vi "HFRR ADV v06 new software.vi"() -> ()   [LabVIEW 2025] (continued)
              n1804 = String Subset(string=w2036, offset (0)=55, length (rest)=9 ("length (rest)")) -> (substring=w2044:string)
              n1805 = String Subset(string=w2036, offset (0)=25) -> (substring=w2040:string)  [unwired: 1 in]
              n1806 = String Subset(string=w2036, offset (0)=15, length (rest)=9 ("length (rest)")) -> (substring=w2065:string)
              n1807 = String Subset(string=w2036, offset (0)=0, length (rest)=14 ("length (rest)")) -> (substring=w2062:string)
              n1808 = String Subset(string=w2036, offset (0)=45, length (rest)=9 ("length (rest)")) -> (substring=w2049:string)
              n1809 = String Subset(string=w2036, offset (0)=65, length (rest)=9 ("length (rest)")) -> (substring=w2055:string)
              n1810 = Fract/Exp String To Number(string=w2038) -> (number=w2035:dbl)  [unwired: 3 in, 1 out]
              n1811 = Fract/Exp String To Number(string=w2059) -> (number=w2057:dbl)  [unwired: 3 in, 1 out]
              n1812 = Fract/Exp String To Number(string=w2044) -> (number=w2042:dbl)  [unwired: 3 in, 1 out]
              n1813 = Fract/Exp String To Number(string=w2040) -> (number=w2039:dbl)  [unwired: 3 in, 1 out]
              n1814 = Fract/Exp String To Number(string=w2065) -> (number=w2056:dbl)  [unwired: 3 in, 1 out]
              n1815 = Fract/Exp String To Number(string=w2062) -> (number=w2058:dbl)  [unwired: 3 in, 1 out]
              n1816 = Fract/Exp String To Number(string=w2049) -> (number=w2046:dbl)  [unwired: 3 in, 1 out]
              n1817 = Fract/Exp String To Number(string=w2055) -> (number=w2052:dbl)  [unwired: 3 in, 1 out]
              n1818 = Add(x=w2052, y=0.0) -> (x+y=w2050:dbl)
            }
            n1819 = String To Path(string=w1895) -> (path=w1993:path)
            n1820 = String To Path(string=w1893) -> (path=w1987:path)
            n1821 = local read "Numeric 11"() -> (w1977:i32)
            n1822 = local read "Numeric 13"() -> (w1979:i32)
            n1823 = Open/Create/Replace File "Open File"(file path (use dialog)=w1993) -> (refnum out=w1991:refnum<file>, error out=w1990:errorcluster)  [unwired: 5 in, 1 out]
            n1824 = Open/Create/Replace File "Open File"(file path (use dialog)=w1987) -> (refnum out=w1986:refnum<file>, error out=w1985:errorcluster)  [unwired: 5 in, 1 out]
            n1825 = for {
              N: w1977 -> [_]
              tunnel: w1991 -> [w2106]
              tunnel: w1990 -> [w2105]
              tunnel: [w2095] -> w1957 mode=indexing
              tunnel: [w2093] -> w1955 mode=indexing
              tunnel: [w2094] -> w1950 mode=indexing
              tunnel: w1976 -> [_]
              tunnel: [w2087] -> w1952 mode=indexing
              tunnel: [w2083] -> w1928 mode=indexing
              tunnel: [w2079] -> w1903 mode=indexing
              tunnel: [w2075] -> w1884 mode=indexing
              tunnel: [w2070] -> w1842 mode=indexing
              (unwired) TRUE ("line mode (F)")
              n1826 = Read from Text File "Read File"(file (use dialog)=w2106, error in=w2105) -> (text=w2071:string)  [unwired: 2 in, 3 out]
              n1827 = local write "String 7"(w2071) -> ()
              n1828 = String Subset(string=w2071, offset (0)=85, length (rest)=9 ("length (rest)")) -> (substring=w2074:string)
              n1829 = String Subset(string=w2071, offset (0)=35, length (rest)=9 ("length (rest)")) -> (substring=w2096:string)
              n1830 = String Subset(string=w2071, offset (0)=55, length (rest)=9 ("length (rest)")) -> (substring=w2082:string)
              n1831 = String Subset(string=w2071, offset (0)=25, length (rest)=9 ("length (rest)")) -> (substring=w2076:string)
              n1832 = String Subset(string=w2071, offset (0)=45, length (rest)=9 ("length (rest)")) -> (substring=w2084:string)
              n1833 = String Subset(string=w2071, offset (0)=0, length (rest)=14 ("length (rest)")) -> (substring=w2099:string)
              n1834 = String Subset(string=w2071, offset (0)=15, length (rest)=9 ("length (rest)")) -> (substring=w2102:string)
              n1835 = String Subset(string=w2071, offset (0)=65, length (rest)=9 ("length (rest)")) -> (substring=w2088:string)
              n1836 = Fract/Exp String To Number(string=w2074) -> (number=w2070:dbl)  [unwired: 3 in, 1 out]
              n1837 = Fract/Exp String To Number(string=w2096) -> (number=w2094:dbl)  [unwired: 3 in, 1 out]
              n1838 = Fract/Exp String To Number(string=w2082) -> (number=w2079:dbl)  [unwired: 3 in, 1 out]
              n1839 = Fract/Exp String To Number(string=w2076) -> (number=w2075:dbl)  [unwired: 3 in, 1 out]
              n1840 = Fract/Exp String To Number(string=w2084) -> (number=w2083:dbl)  [unwired: 3 in, 1 out]
              n1841 = Fract/Exp String To Number(string=w2099) -> (number=w2095:dbl)  [unwired: 3 in, 1 out]
              n1842 = Fract/Exp String To Number(string=w2102) -> (number=w2093:dbl)  [unwired: 3 in, 1 out]
              n1843 = Fract/Exp String To Number(string=w2088) -> (number=w2091:dbl)  [unwired: 3 in, 1 out]
              n1844 = Add(x=w2091, y=0.0) -> (x+y=w2087:dbl)
            }
            n1845 = for {
              N: w1979 -> [_]
              tunnel: w1986 -> [w2034]
              tunnel: w1985 -> [w2033]
              tunnel: [w2023] -> w1939 mode=indexing
              tunnel: [w2022] -> w1932 mode=indexing
              tunnel: w1976 -> [_]
              tunnel: [w2011] -> w1937 mode=indexing
              tunnel: [w2016] -> w1934 mode=indexing
              tunnel: [w2012] -> w1924 mode=indexing
              tunnel: [w2007] -> w1899 mode=indexing
              tunnel: [w2003] -> w1880 mode=indexing
              tunnel: [w1998] -> w1840 mode=indexing
              (unwired) 1.0 ("x")
              (unwired) TRUE ("line mode (F)")
              n1846 = Read from Text File "Read File"(file (use dialog)=w2034, error in=w2033) -> (text=w1999:string)  [unwired: 2 in, 3 out]
              n1847 = local write "String 12"(w1999) -> ()
              n1848 = String Subset(string=w1999, offset (0)=85, length (rest)=9 ("length (rest)")) -> (substring=w2001:string)
              n1849 = String Subset(string=w1999, offset (0)=35, length (rest)=9 ("length (rest)")) -> (substring=w2024:string)
              n1850 = String Subset(string=w1999, offset (0)=55, length (rest)=9 ("length (rest)")) -> (substring=w2009:string)
              n1851 = String Subset(string=w1999, offset (0)=25, length (rest)=9 ("length (rest)")) -> (substring=w2005:string)
              n1852 = String Subset(string=w1999, offset (0)=45, length (rest)=9 ("length (rest)")) -> (substring=w2014:string)
              n1853 = String Subset(string=w1999, offset (0)=15, length (rest)=9 ("length (rest)")) -> (substring=w2030:string)
              n1854 = String Subset(string=w1999, offset (0)=0, length (rest)=14 ("length (rest)")) -> (substring=w2027:string)
              n1855 = String Subset(string=w1999, offset (0)=65, length (rest)=9 ("length (rest)")) -> (substring=w2017:string)
              n1856 = Fract/Exp String To Number(string=w2001) -> (number=w1998:dbl)  [unwired: 3 in, 1 out]
              n1857 = Fract/Exp String To Number(string=w2024) -> (number=w2022:dbl)  [unwired: 3 in, 1 out]
              n1858 = Fract/Exp String To Number(string=w2009) -> (number=w2007:dbl)  [unwired: 3 in, 1 out]
              n1859 = Fract/Exp String To Number(string=w2005) -> (number=w2003:dbl)  [unwired: 3 in, 1 out]
              n1860 = Fract/Exp String To Number(string=w2014) -> (number=w2012:dbl)  [unwired: 3 in, 1 out]
              n1861 = Fract/Exp String To Number(string=w2030) -> (number=w2011:dbl)  [unwired: 3 in, 1 out]
              n1862 = Fract/Exp String To Number(string=w2027) -> (number=w2023:dbl)  [unwired: 3 in, 1 out]
              n1863 = Fract/Exp String To Number(string=w2017) -> (number=w2020:dbl)  [unwired: 3 in, 1 out]
              n1864 = Add(x=w2020, y=0.0) -> (x+y=w2016:dbl)
            }
            n1865 = Delete From Array(array=w1882, index=0) -> (array with subset deleted=w1855:dbl[])  [unwired: 1 in, 1 out]
            n1866 = Delete From Array(array=w1945, index=0) -> (array with subset deleted=w1918:dbl[])  [unwired: 1 in, 1 out]
            n1867 = Delete From Array(array=w1925, index=0) -> (array with subset deleted=w1913:dbl[])  [unwired: 1 in, 1 out]
            n1868 = Delete From Array(array=w1943, index=0) -> (array with subset deleted=w1944:dbl[])  [unwired: 1 in, 1 out]
            n1869 = call-poly <vilib>:"Mean.vi"("X"=w1855) -> ("mean"=→"КОФ2 4":dbl)  [unwired: 1 out]
            n1870 = call-poly <vilib>:"Mean.vi"("X"=w1918) -> ("mean"=→"КОФ3":dbl)  [unwired: 1 out]
            n1871 = call-poly <vilib>:"Mean.vi"("X"=w1913) -> ("mean"=→"CP3":dbl)  [unwired: 1 out]
            n1872 = Delete From Array(array=w1907, index=0) -> (array with subset deleted=w1834:dbl[])  [unwired: 1 in, 1 out]
            n1873 = Delete From Array(array=w1846, index=0) -> (array with subset deleted=w1833:dbl[])  [unwired: 1 in, 1 out]
            n1874 = Delete From Array(array=w1886, index=0) -> (array with subset deleted=w1857:dbl[])  [unwired: 1 in, 1 out]
            n1875 = Delete From Array(array=w1964, index=0) -> (array with subset deleted=w1919:dbl[])  [unwired: 1 in, 1 out]
            n1876 = Delete From Array(array=w1930, index=0) -> (array with subset deleted=w1915:dbl[])  [unwired: 1 in, 1 out]
            "array w/ subset deleted" <- w1915
            n1877 = Delete From Array(array=w1961, index=0) -> (array with subset deleted=w1962:dbl[])  [unwired: 1 in, 1 out]
            n1878 = call-poly <vilib>:"Mean.vi"("X"=w1857) -> ("mean"=→"КОФ2 2":dbl)  [unwired: 1 out]
            n1879 = call-poly <vilib>:"Mean.vi"("X"=w1919) -> ("mean"=→"КОФ1":dbl)  [unwired: 1 out]
            n1880 = Bundle "Bundle"(w1834, w1833) -> (w1839:cluster{dbl[], dbl[]})  [unwired: 1 in]
            n1881 = Bundle "Bundle"(w1834, w1962) -> (w1826:cluster{dbl[], dbl[]})  [unwired: 1 in]
            n1882 = Delete From Array(array=w1841, index=0) -> (array with subset deleted=w1829:dbl[])  [unwired: 1 in, 1 out]
            n1883 = Delete From Array(array=w1842, index=0) -> (array with subset deleted=w1831:dbl[])  [unwired: 1 in, 1 out]
            n1884 = Delete From Array(array=w1952, index=0) -> (array with subset deleted=w1953:dbl[])  [unwired: 1 in, 1 out]
            n1885 = Delete From Array(array=w1840, index=0) -> (array with subset deleted=w1827:dbl[])  [unwired: 1 in, 1 out]
            n1886 = Delete From Array(array=w1934, index=0) -> (array with subset deleted=w1935:dbl[])  [unwired: 1 in, 1 out]
            n1887 = Delete From Array(array=w1959, index=0) -> (array with subset deleted=w1865:dbl[])  [unwired: 1 in, 1 out]
            n1888 = Delete From Array(array=w1905, index=0) -> (array with subset deleted=w1861:dbl[])  [unwired: 1 in, 1 out]
            n1889 = Delete From Array(array=w1941, index=0) -> (array with subset deleted=w1863:dbl[])  [unwired: 1 in, 1 out]
            n1890 = Delete From Array(array=w1901, index=0) -> (array with subset deleted=w1859:dbl[])  [unwired: 1 in, 1 out]
            n1891 = Delete From Array(array=w1950, index=0) -> (array with subset deleted=w1864:dbl[])  [unwired: 1 in, 1 out]
            n1892 = Delete From Array(array=w1903, index=0) -> (array with subset deleted=w1860:dbl[])  [unwired: 1 in, 1 out]
            n1893 = Delete From Array(array=w1884, index=0) -> (array with subset deleted=w1856:dbl[])  [unwired: 1 in, 1 out]
            n1894 = Delete From Array(array=w1928, index=0) -> (array with subset deleted=w1914:dbl[])  [unwired: 1 in, 1 out]
            n1895 = Delete From Array(array=w1955, index=0) -> (array with subset deleted=w1916:dbl[])  [unwired: 1 in, 1 out]
            n1896 = Delete From Array(array=w1932, index=0) -> (array with subset deleted=w1862:dbl[])  [unwired: 1 in, 1 out]
            n1897 = Delete From Array(array=w1899, index=0) -> (array with subset deleted=w1858:dbl[])  [unwired: 1 in, 1 out]
            n1898 = Delete From Array(array=w1880, index=0) -> (array with subset deleted=w1854:dbl[])  [unwired: 1 in, 1 out]
            n1899 = Delete From Array(array=w1924, index=0) -> (array with subset deleted=w1912:dbl[])  [unwired: 1 in, 1 out]
            n1900 = Delete From Array(array=w1937, index=0) -> (array with subset deleted=w1917:dbl[])  [unwired: 1 in, 1 out]
            n1901 = Delete From Array(array=w1947, index=0) -> (array with subset deleted=w1830:dbl[])  [unwired: 1 in, 1 out]
            n1902 = Delete From Array(array=w1957, index=0) -> (array with subset deleted=w1832:dbl[])  [unwired: 1 in, 1 out]
            n1903 = Delete From Array(array=w1939, index=0) -> (array with subset deleted=w1828:dbl[])  [unwired: 1 in, 1 out]
            n1904 = Bundle "Bundle"(w1834, w1865) -> (w1852:cluster{dbl[], dbl[]})  [unwired: 1 in]
            n1905 = Bundle "Bundle"(w1834, w1919) -> (w1853:cluster{dbl[], dbl[]})  [unwired: 1 in]
            n1906 = Bundle "Bundle"(w1865, w1861) -> (w1867:cluster{dbl[], dbl[]})  [unwired: 1 in]
            n1907 = Bundle "Bundle"(w1830, w1829) -> (w1837:cluster{dbl[], dbl[]})  [unwired: 1 in]
            n1908 = Bundle "Bundle"(w1863, w1859) -> (w1869:cluster{dbl[], dbl[]})  [unwired: 1 in]
            n1909 = Bundle "Bundle"(w1830, w1863) -> (w1973:cluster{dbl[], dbl[]})  [unwired: 1 in]
            n1910 = Bundle "Bundle"(w1830, w1859) -> (w1897:cluster{dbl[], dbl[]})  [unwired: 1 in]
            n1911 = Bundle "Bundle"(w1830, w1918) -> (w1983:cluster{dbl[], dbl[]})  [unwired: 1 in]
            n1912 = Bundle "Bundle"(w1830, w1913) -> (w1921:cluster{dbl[], dbl[]})  [unwired: 1 in]
            n1913 = Bundle "Bundle"(w1830, w1944) -> (w1968:cluster{dbl[], dbl[]})  [unwired: 1 in]
            n1914 = Bundle "Bundle"(w1864, w1860) -> (w1868:cluster{dbl[], dbl[]})  [unwired: 1 in]
            n1915 = Bundle "Bundle"(w1832, w1831) -> (w1838:cluster{dbl[], dbl[]})  [unwired: 1 in]
            n1916 = Bundle "Bundle"(w1832, w1864) -> (w1975:cluster{dbl[], dbl[]})  [unwired: 1 in]
            n1917 = Bundle "Bundle"(w1832, w1860) -> (w1898:cluster{dbl[], dbl[]})  [unwired: 1 in]
            n1918 = Bundle "Bundle"(w1832, w1914) -> (w1922:cluster{dbl[], dbl[]})  [unwired: 1 in]
            n1919 = Bundle "Bundle"(w1832, w1916) -> (w1984:cluster{dbl[], dbl[]})  [unwired: 1 in]
            n1920 = Bundle "Bundle"(w1832, w1953) -> (w1966:cluster{dbl[], dbl[]})  [unwired: 1 in]
            n1921 = Bundle "Bundle"(w1862, w1858) -> (w1870:cluster{dbl[], dbl[]})  [unwired: 1 in]
            n1922 = Bundle "Bundle"(w1828, w1827) -> (w1836:cluster{dbl[], dbl[]})  [unwired: 1 in]
            n1923 = Bundle "Bundle"(w1828, w1862) -> (w1974:cluster{dbl[], dbl[]})  [unwired: 1 in]
            n1924 = Bundle "Bundle"(w1828, w1858) -> (w1896:cluster{dbl[], dbl[]})  [unwired: 1 in]
            n1925 = Bundle "Bundle"(w1828, w1912) -> (w1920:cluster{dbl[], dbl[]})  [unwired: 1 in]
            n1926 = Bundle "Bundle"(w1828, w1917) -> (w1982:cluster{dbl[], dbl[]})  [unwired: 1 in]
            n1927 = Bundle "Bundle"(w1828, w1935) -> (w1967:cluster{dbl[], dbl[]})  [unwired: 1 in]
            n1928 = call-poly <vilib>:"Mean.vi"("X"=w1915) -> ("mean"=→"CP1":dbl)  [unwired: 1 out]
            n1929 = call-poly <vilib>:"Mean.vi"("X"=w1856) -> ("mean"=→"КОФ2 3":dbl)  [unwired: 1 out]
            n1930 = call-poly <vilib>:"Mean.vi"("X"=w1914) -> ("mean"=→"CP2":dbl)  [unwired: 1 out]
            n1931 = call-poly <vilib>:"Mean.vi"("X"=w1916) -> ("mean"=→"КОФ2":dbl)  [unwired: 1 out]
            n1932 = call-poly <vilib>:"Mean.vi"("X"=w1854) -> ("mean"=→"КОФ2 5":dbl)  [unwired: 1 out]
            n1933 = call-poly <vilib>:"Mean.vi"("X"=w1912) -> ("mean"=→"CP4":dbl)  [unwired: 1 out]
            n1934 = call-poly <vilib>:"Mean.vi"("X"=w1917) -> ("mean"=→"КОФ4":dbl)  [unwired: 1 out]
            n1935 = Bundle "Bundle"(w1834, w1861) -> (w1825:cluster{dbl[], dbl[]})  [unwired: 1 in]
            n1936 = Bundle "Bundle"(w1834, w1915) -> (w1848:cluster{dbl[], dbl[]})  [unwired: 1 in]
            n1937 = Build Array "Build Array"(w1825, w1848) -> (w1851:cluster{dbl[], dbl[]}[])
            "XY Graph 17" <- w1851
            n1938 = Build Array "Build Array"(w1839, w1838, w1837, w1836) -> (→"Frequency ( Hz )":cluster{dbl[], dbl[]}[])
            n1939 = Build Array "Build Array"(w1867, w1868, w1869, w1870) -> (→"Air Temp ( °C ) vs Humidity ( % RH )":cluster{dbl[], dbl[]}[])
            n1940 = Build Array "Build Array"(w1852, w1975, w1973, w1974) -> (→"Air Temperature  ( °C )":cluster{dbl[], dbl[]}[])
            n1941 = Build Array "Build Array"(w1825, w1898, w1897, w1896) -> (→"Humidity ( %RH )":cluster{dbl[], dbl[]}[])
            n1942 = Build Array "Build Array"(w1853, w1984, w1983, w1982) -> (→"Coefficient Of Friction":cluster{dbl[], dbl[]}[])
            n1943 = Build Array "Build Array"(w1848, w1922, w1921, w1920) -> (→"Sample Temperature ( °C )":cluster{dbl[], dbl[]}[])
            n1944 = Build Array "Build Array"(w1826, w1966, w1968, w1967) -> (→"XY Graph 13":cluster{dbl[], dbl[]}[])
            n1945 = Bundle "Bundle"(w1834, w1857) -> (w1879:cluster{dbl[], dbl[]})  [unwired: 1 in]
            n1946 = Bundle "Bundle"(w1830, w1855) -> (w1877:cluster{dbl[], dbl[]})  [unwired: 1 in]
            n1947 = Bundle "Bundle"(w1832, w1856) -> (w1878:cluster{dbl[], dbl[]})  [unwired: 1 in]
            n1948 = Bundle "Bundle"(w1828, w1854) -> (w1876:cluster{dbl[], dbl[]})  [unwired: 1 in]
            n1949 = Build Array "Build Array"(w1879, w1878, w1877, w1876) -> (→"Stroke ( mm )":cluster{dbl[], dbl[]}[])
            n1950 = local write "XY Graph 16"(w1851) -> ()
          }
          frame #2 {
          }
          frame #3 {
            n1951 = local write "Numeric 8"(0 ("Numeric 8")) -> ()
            n1952 = local write "Numeric 11"(0 ("Numeric 11")) -> ()
            n1953 = local write "Numeric 12"(0 ("Numeric 12")) -> ()
            n1954 = local write "Numeric 13"(0 ("Numeric 13")) -> ()
            n1955 = property on="OPEN" class="Bool (strict)"("Visible"=TRUE) -> ()  [unwired: 2 in, 2 out]
            n1956 = local read "String Control 2"() -> (w2151:string)
            n1957 = local read "String Control 4"() -> (w2150:string)
            n1958 = local read "String Control 6"() -> (w2149:string)
            n1959 = local read "String Control 8"() -> (w2148:string)
            n1960 = Match Pattern(string=w2151, regular expression="Samples / cycle :- ") -> (after substring=w2165:string)  [unwired: 1 in, 3 out]
            n1961 = Match Pattern(string=w2151, regular expression="Frequency :- ") -> (after substring=w2184:string)  [unwired: 1 in, 3 out]
            n1962 = Match Pattern(string=w2150, regular expression="Samples / cycle :- ") -> (after substring=w2161:string)  [unwired: 1 in, 3 out]
            n1963 = Match Pattern(string=w2150, regular expression="Frequency :- ") -> (after substring=w2179:string)  [unwired: 1 in, 3 out]
            n1964 = Match Pattern(string=w2149, regular expression="Samples / cycle :- ") -> (after substring=w2157:string)  [unwired: 1 in, 3 out]
            n1965 = Match Pattern(string=w2149, regular expression="Frequency :- ") -> (after substring=w2174:string)  [unwired: 1 in, 3 out]
            n1966 = Match Pattern(string=w2148, regular expression="Samples / cycle :- ") -> (after substring=w2153:string)  [unwired: 1 in, 3 out]
            n1967 = Match Pattern(string=w2148, regular expression="Frequency :- ") -> (after substring=w2169:string)  [unwired: 1 in, 3 out]
            n1968 = String Subset(string=w2165, length (rest)=6 ("length (rest)")) -> (substring=w2167:string)  [unwired: 1 in]
            n1969 = String Subset(string=w2184, length (rest)=9 ("length (rest)")) -> (substring=w2186:string)  [unwired: 1 in]
            n1970 = String Subset(string=w2161, length (rest)=6 ("length (rest)")) -> (substring=w2163:string)  [unwired: 1 in]
            n1971 = String Subset(string=w2179, length (rest)=9 ("length (rest)")) -> (substring=w2181:string)  [unwired: 1 in]
            n1972 = String Subset(string=w2157, length (rest)=6 ("length (rest)")) -> (substring=w2159:string)  [unwired: 1 in]
            n1973 = String Subset(string=w2174, length (rest)=9 ("length (rest)")) -> (substring=w2176:string)  [unwired: 1 in]
            n1974 = String Subset(string=w2153, length (rest)=6 ("length (rest)")) -> (substring=w2155:string)  [unwired: 1 in]
            n1975 = String Subset(string=w2169, length (rest)=9 ("length (rest)")) -> (substring=w2171:string)  [unwired: 1 in]
            n1976 = Fract/Exp String To Number(string=w2167) -> (number=w2147:dbl)  [unwired: 3 in, 1 out]
            n1977 = Fract/Exp String To Number(string=w2186) -> (number=w2187:dbl)  [unwired: 3 in, 1 out]
            n1978 = Fract/Exp String To Number(string=w2163) -> (number=w2146:dbl)  [unwired: 3 in, 1 out]
            n1979 = Fract/Exp String To Number(string=w2181) -> (number=w2182:dbl)  [unwired: 3 in, 1 out]
            n1980 = Fract/Exp String To Number(string=w2159) -> (number=w2145:dbl)  [unwired: 3 in, 1 out]
            n1981 = Fract/Exp String To Number(string=w2176) -> (number=w2177:dbl)  [unwired: 3 in, 1 out]
            n1982 = Fract/Exp String To Number(string=w2155) -> (number=w2144:dbl)  [unwired: 3 in, 1 out]
            n1983 = Fract/Exp String To Number(string=w2171) -> (number=w2172:dbl)  [unwired: 3 in, 1 out]
            n1984 = local write "sample1"(w2147) -> ()
            n1985 = local write "freq1"(w2187) -> ()
            n1986 = local write "sample2"(w2146) -> ()
            n1987 = local write "freq2"(w2182) -> ()
            n1988 = local write "sample3"(w2145) -> ()
            n1989 = local write "freq3"(w2177) -> ()
            n1990 = local write "sample4"(w2144) -> ()
            n1991 = local write "freq 4"(w2172) -> ()
          }
        }
      }
    }
    n1992 = case shown="True" w1636 {
      selector: w1636 -> [_ w1764]
      frame False {
      }
      frame True {
        n1993 = Not(x=w1764) -> (.not. x?=w1760:bool)
        n1994 = local write "service 3"(w1760) -> ()
        n1995 = local write "OPEN 6"(w1760) -> ()
        n1996 = call <vilib>:"System Exec.vi"("wait until completion? (T)"=TRUE, "command line"="C:\\LAB-IQ\\Scar View.exe") -> ("error out"=→"error out 5":errorcluster)  [unwired: 6 in, 3 out]
      }
    }
    n1997 = case shown="\"Acquire\", Default" w1647 {
      frame "Acquire", Default {
        w2660 = 0.2 ("y")
        w2665 = 1.0 ("y")
        w2666 = 0.8 ("y")
        # "Elapsed time\ncof\nstroke\nAir temp\nTemp\nHumidity"
        n1998 = disable-structure shown="Disabled" {
          frame Disabled {
            n1999 = local read "Flag"() -> (w2683:dbl)
            n2000 = local read "RUN"() -> (w2680:bool)
            n2001 = Not(x=w2680) -> (.not. x?=w2679:bool)
            n2002 = Equal?(x=w2683, y=10.0) -> (x = y?=w2681:bool)
            n2003 = And(x=w2681, y=w2679) -> (x .and. y?=w2678:bool)
            n2004 = case shown="True" w2678 {
              frame False {
              }
              frame True {
                w2684 = FALSE ("Heater Button")
                n2005 = local write "Humidity"(w2684) -> ()
                n2006 = local write "Heater Button"(w2684) -> ()
              }
            }
          }
          frame Enabled {
          }
        }
        n2007 = disable-structure shown="Disabled" {
          frame Disabled {
            n2008 = case shown="True" {
              selector: _ -> [_ _]
              frame False {
              }
              frame True {
                w2775 = TRUE ("Heater")
                n2009 = local write "Humidity"(w2775) -> ()
                n2010 = local write "Heater Button"(w2775) -> ()
                n2011 = local read "TEST STANDARD"() -> (w2778:T3)
                n2012 = local read "TEST STANDARD"() -> (w2773:T3)
                n2013 = Equal?(x=w2778, y=enum16{"ASTM D6079", "ISO 12156", "Custom"}."ISO 12156" ("Test Standard")) -> (x = y?=w2776:bool)
                n2014 = Equal?(x=w2773, y=enum16{"ASTM D6079", "ISO 12156", "Custom"}."ASTM D6079" ("Test Standard")) -> (x = y?=w2772:bool)
                n2015 = case shown="True" w2776 {
                  frame False {
                  }
                  frame True {
                    n2016 = local write "Heater"(TRUE ("Heater")) -> ()
                    n2017 = local write "airtempflg"(FALSE ("airtempflg")) -> ()
                  }
                }
                n2018 = case shown="True" w2772 {
                  frame False {
                  }
                  frame True {
                    n2019 = local write "Heater"(FALSE ("Heater")) -> ()
                    n2020 = local write "airtempflg"(TRUE ("airtempflg")) -> ()
                  }
                }
              }
            }
          }
          frame Enabled {
          }
        }
        n2021 = stacked-sequence {
          frame #0 {
            n2022 = case shown="True" "RST FF" {
              frame False {
              }
              frame True {
                w2841 = 0.0 ("X Scale.Range:Maximum")
                n2023 = property on="Frictional Force ( N )" class="WFChart (strict)"("XScale.Maximum"=600.0 ("X Scale.Range:Maximum"), "XScale.Minimum"=w2841, "YScale.Maximum"=10.0 ("Y Scale.Range:Maximum"), "YScale.Minimum"=w2841) -> ()  [unwired: 2 in, 2 out]
              }
            }
          }
          frame #1 {
            n2024 = case shown="True" "RST TEMP" {
              frame False {
              }
              frame True {
                n2025 = property on="Temperature ( Deg C )" class="WFChart (strict)"("XScale.Minimum"=0.0 ("X Scale.Range:Minimum"), "XScale.Maximum"=600.0 ("X Scale.Range:Maximum"), "YScale.Minimum"=0.0 ("Y Scale.Range:Minimum"), "YScale.Maximum"=100.0 ("Y Scale.Range:Maximum")) -> ()  [unwired: 2 in, 2 out]
              }
            }
          }
          frame #2 {
            n2026 = case shown="True" "RSTCOF" {
              frame False {
              }
              frame True {
                n2027 = property on="Coefficient of Friction" class="WFChart (strict)"("XScale.Minimum"=0.0 ("X Scale.Range:Minimum"), "XScale.Maximum"=600.0 ("X Scale.Range:Maximum"), "YScale.Maximum"=1.0 ("X Scale.Range:Minimum"), "YScale.Minimum"=0.0 ("X Scale.Range:Minimum")) -> ()  [unwired: 2 in, 2 out]
              }
            }
          }
          frame #3 {
            n2028 = case shown="True" "RSTCOF 2" {
              frame False {
              }
              frame True {
                (unwired) 100.0 ("Y Scale.Range:Maximum")
                (unwired) 0.0 ("Y Scale.Range:Minimum")
                (unwired) 600.0 ("X Scale.Range:Maximum")
                (unwired) 0.0 ("X Scale.Range:Minimum")
              }
            }
          }
          frame #4 {
            n2029 = case shown="True" "RSTCOF 3" {
              frame False {
              }
              frame True {
                n2030 = property on="Electrical Contact Resistance ( % )" class="WFChart (strict)"("XScale.Minimum"=0.0 ("X Scale.Range:Minimum"), "XScale.Maximum"=600.0 ("X Scale.Range:Maximum"), "YScale.Minimum"=0.0 ("Y Scale.Range:Minimum"), "YScale.Maximum"=100.0 ("Y Scale.Range:Maximum")) -> ()  [unwired: 2 in, 2 out]
              }
            }
          }
        }
        n2031 = disable-structure shown="Disabled" {
          frame Disabled {
            n2032 = case shown="True" {
              selector: _ -> [_ _]
              frame False {
              }
              frame True {
                n2033 = local read "zflag 2"() -> (w2742:dbl)
                n2034 = local read "yflag"() -> (w2744:dbl)
                n2035 = Equal?(x=w2744, y=2.0 ("tflag")) -> (x = y?=w2746:bool)
                n2036 = Equal?(x=w2742, y=3.0 ("tflag")) -> (x = y?=w2745:bool)
                n2037 = And(x=w2746, y=w2745) -> (x .and. y?=w2740:bool)
                n2038 = case shown="True" w2740 {
                  frame False {
                  }
                  frame True {
                    w2771 = 0.0 ("zflag")
                    n2039 = local write "zflag"(w2771) -> ()
                    n2040 = local write "zflag 2"(w2771) -> ()
                    n2041 = Delete(path (use dialog)=path "C:/LAB-IQ-NXT/WO 2449 TT.sig" ("file path (dialog if empty)")) -> (deleted path=w2770:path)  [unwired: 4 in, 2 out]
                    n2042 = Delete(path (use dialog)=path "C:/LAB-IQ-NXT/WO 2449 TRH.sig" ("file path (dialog if empty)")) -> (deleted path=w2765:path)  [unwired: 4 in, 2 out]
                    n2043 = local read "SEN.RUN HRS"() -> (w2757:dbl)
                    n2044 = local read "SENSOR TIME"() -> (w2755:dbl)
                    n2045 = call <vilib>:"compatOverwrite.vi"("overwrite (F)"=TRUE) -> ("overwrite?"=w2747:T25)
                    n2046 = call <vilib>:"compatOverwrite.vi"("overwrite (F)"=TRUE) -> ("overwrite?"=w2751:T25)
                    n2047 = local read "Total No. of Tests"() -> (w2758:dbl)
                    n2048 = Add(x=w2755, y=w2757) -> (x+y=w2756:dbl)
                    "SEN.RUN HRS" <- w2756
                    n2049 = Open/Create/Replace File(file path (use dialog)=w2770, operation (0:open)=w2747) -> (refnum out=w2748:refnum<file>, error out=w2749:errorcluster)  [unwired: 4 in, 1 out]
                    n2050 = Open/Create/Replace File(file path (use dialog)=w2765, operation (0:open)=w2751) -> (refnum out=w2752:refnum<file>, error out=w2753:errorcluster)  [unwired: 4 in, 1 out]
                    n2051 = Deny Access(4:w2749, 6:T23."deny none" ("deny mode (2)"), 7:w2748) -> (3:w2769:refnum<file>)  [unwired: 1 out]
                    n2052 = Deny Access(4:w2753, 6:T23."deny none" ("deny mode (2)"), 7:w2752) -> (3:w2761:refnum<file>)  [unwired: 1 out]
                    n2053 = Number To Decimal String(number=w2758) -> (decimal integer string=w2766:string)  [unwired: 1 in]
                    n2054 = Number To Decimal String(number=w2756) -> (decimal integer string=w2762:string)  [unwired: 1 in]
                    n2055 = Write to Binary File(file (use dialog)=w2769, data=w2766, 5:FALSE ("prepend array or string size? (T)")) -> ()  [unwired: 3 in, 3 out]
                    n2056 = Write to Binary File(file (use dialog)=w2761, data=w2762, 5:FALSE ("prepend array or string size? (T)")) -> ()  [unwired: 3 in, 3 out]
                  }
                }
              }
            }
          }
          frame Enabled {
          }
        }
        n2057 = local read "RUN"() -> (w2669:bool)
        n2058 = local read "run replace"() -> (w2673:bool)
        n2059 = local read "run replace"() -> (w2672:bool)
        n2060 = case shown="True" w2669 {
          frame False {
            n2061 = local write "run replace"(FALSE ("run replace")) -> ()
          }
          frame True {
            "run replace" <- TRUE ("run replace")
          }
        }
        n2062 = local read "RUN"() -> (w2677:bool)
        n2063 = local read "Set Temp"() -> (w2639:dbl)
        n2064 = local read "SetTemp"() -> (w2641:dbl)
        n2065 = case shown="False" w2677 {
          tunnel: [FALSE ("TEST RUNNING") TRUE ("TEST RUNNING")] -> w2676
          frame False {
            w2860 = 0.0 ("Flag")
            n2066 = local write "Elapsed time"(0.0 ("elapsedtime")) -> ()
            n2067 = local write "Time Remaining"(w2860) -> ()
            n2068 = local write "Flag"(w2860) -> ()
            n2069 = local write "Remaining Time"(w2860) -> ()
          }
          frame True {
            n2070 = local write "Flag"(10.0 ("Flag")) -> ()
          }
        }
        n2071 = case shown="False" w2673 {
          frame False {
            n2072 = local read "zflag"() -> (→"zflag 2":dbl)
            n2073 = local write "yflag"(2.0 ("tflag")) -> ()
            n2074 = local write "FLAG 4"(0.0 ("FLAG")) -> ()
          }
          frame True {
            n2075 = local write "yflag"(1.0 ("tflag")) -> ()
            n2076 = local write "zflag"(3.0 ("zflag")) -> ()
          }
        }
        n2077 = local read "acq 2"() -> (w2671:bool)
        n2078 = local read "AIR TEMP"() -> (w2634:dbl)
        n2079 = local read "Amb temp"() -> (w2638:dbl)
        n2080 = case shown="True" "Save & Continue" {
          frame False {
          }
          frame True {
            "acq 2" <- TRUE ("acq 2")
          }
        }
        n2081 = local read "Set Rh"() -> (w2640:dbl)
        n2082 = Add(x=w2641, y=w2666) -> (x+y=w2667:dbl)
        n2083 = Subtract(x=w2641, y=w2666) -> (x-y=w2668:dbl)
        n2084 = Add(x=w2639, y=w2660) -> (x+y=w2661:dbl)
        n2085 = Subtract(x=w2639, y=w2660) -> (x-y=w2662:dbl)
        n2086 = And(x=w2671, y=w2672) -> (x .and. y?=w2670:bool)
        n2087 = Greater Or Equal?(x=w2634, y=15.0) -> (x >= y?=w2635:bool)
        "powstat" <- w2635
        n2088 = local read "Humidity ( %RH )"() -> (w2637:dbl)
        n2089 = case shown="True" "Save & Continue" {
          frame False {
          }
          frame True {
            n2090 = while {
              tunnel: "0123456789abcdefghijklmnopqrstuvwxyzABCDEFGHIJKLMNOPQRSTUVWXYZ" ("string 2") -> [w2831]
              shift-right: [w2829] -> w2824
              shift-left: "" -> [w2828]
              i -> [w2838]
              stop <- w2837 stop-if-true
              n2091 = Random Number (0-1)() -> (number: 0 to 1=w2832:dbl)
              n2092 = Multiply(x=w2832, y=62.0) -> (x*y=w2834:dbl)
              n2093 = Decrement(x="Length") -> (x-1=w2827:i16)
              n2094 = To Word Integer(number=w2834) -> (16bit integer=w2835:i16)
              n2095 = String Subset(string=w2831, offset (0)=w2835, length (rest)=1 ("length (rest)")) -> (substring=w2830:string)
              n2096 = Greater Or Equal?(x=w2838, y=w2827) -> (x >= y?=w2837:bool)
              n2097 = Concatenate Strings(w2830, w2828) -> (w2829:string)
            }
            n2098 = local write "UUID"(w2824) -> ()
          }
        }
        n2099 = In Range and Coerce(upper limit=w2667, x=w2638, lower limit=w2668) -> (In Range?=w2657:bool)  [unwired: 1 out]
        n2100 = Add(x=w2640, y=w2665) -> (x+y=w2664:dbl)
        n2101 = Subtract(x=w2640, y=w2665) -> (x-y=w2663:dbl)
        n2102 = local read "TEMP"() -> (w2636:dbl)
        n2103 = case shown="True" "Save & Continue" {
          frame False {
          }
          frame True {
            n2104 = local read "Operator ID"() -> (w3148:string)
            n2105 = local read "FILE"() -> (w3154:string)
            n2106 = String Length(string=w3154) -> (length=w3152:i32)
            n2107 = String Length(string=w3148) -> (length=w3149:i32)
            n2108 = Greater?(x=w3152, y=0) -> (0:w3151:bool)
            n2109 = Greater?(x=w3149, y=0) -> (0:w3147:bool)
            n2110 = And(x=w3151, y=w3147) -> (x .and. y?=w3146:bool)
            n2111 = case shown="True" w3146 {
              frame False {
                n2112 = stacked-sequence {
                  frame #0 {
                    n2113 = One Button Dialog(message="Please Enter a File Name and Operator ID to save data !", button name ("OK")="Ok") -> ()  [unwired: 1 out]
                  }
                  frame #1 {
                    n2114 = local write "Save & Continue"(FALSE ("OK Button")) -> ()
                  }
                }
                n2115 = local write "Save & Continue"(FALSE ("OK Button")) -> ()
              }
              frame True {
                n2116 = stacked-sequence {
                  frame #0 {
                    n2117 = local read "FILE"() -> (w3160:string)
                    n2118 = call "file check.vi"("file name in"=w3160) -> ("file name out"=w3159:string)  [unwired: 9 in, 1 out]
                    n2119 = call <vilib>:"Application Directory.vi"() -> ("Application Directory"=w3170:path)
                    n2120 = Build Path(base path=w3170, name or relative path="data") -> (appended path=w3169:path)
                    n2121 = call <vilib>:"Trim Whitespace.vi"("string"=w3159) -> ("trimmed string"=w3167:string)  [unwired: 1 in]
                    n2122 = call <vilib>:"Trim Whitespace.vi"("string"=w3159) -> ("trimmed string"=w3168:string)  [unwired: 1 in]
                    n2123 = List Folder(path=w3169) -> (folder names=w3165:string[])  [unwired: 3 in, 3 out]
                    n2124 = Match Pattern(string=w3167, regular expression="_(") -> (before substring=w3164:string)  [unwired: 1 in, 3 out]
                    n2125 = for {
                      tunnel: w3165 -> [w3179] mode=indexing
                      tunnel: w3164 -> [w3177]
                      shift-right: [w3175] -> w3162
                      shift-left: bool[] [] -> [w3176]
                      n2126 = Match Pattern(string=w3179, regular expression="_(") -> (before substring=w3178:string)  [unwired: 1 in, 3 out]
                      n2127 = Equal?(x=w3178, y=w3177) -> (x = y?=w3174:bool)
                      n2128 = case shown="True" w3174 {
                        tunnel: w3174 -> [_ w3182]
                        tunnel: w3176 -> [w3181 w3184]
                        tunnel: [w3181 w3183] -> w3175
                        frame False {
                        }
                        frame True {
                          n2129 = Insert Into Array(array=w3184, new element=w3182) -> (w3183:bool[])  [unwired: 1 in]
                        }
                      }
                    }
                    n2130 = Equal?(x=w3165, y=w3164) -> (x = y?=w3173:bool[])
                    n2131 = Or Array Elements(Boolean array=w3173) -> (logical OR=w3172:bool)
                    n2132 = Array Size(array=w3162) -> (size(s)=w3161:i32)
                    n2133 = case shown="True" w3172 {
                      tunnel: w3168 -> [_ w3192]
                      tunnel: w3161 -> [_ w3185]
                      frame False {
                      }
                      frame True {
                        n2134 = Number To Decimal String(number=w3185) -> (decimal integer string=w3188:string)  [unwired: 1 in]
                        n2135 = Search/Split String(string=w3192, search string/char (-)="_(" ("regular expression")) -> (substring before match=w3190:string)  [unwired: 1 in, 2 out]
                        n2136 = Concatenate Strings(w3190, "_(" ("regular expression"), w3188, ")" ("regular expression")) -> (w3186:string)
                        n2137 = local write "FILE"(w3186) -> ()
                      }
                    }
                  }
                  frame #1 {
                    w3194 = 0.0
                    w3207 = cluster{"y":dbl, dbl, "y":dbl}[] [] ("History Data")
                    w3208 = FALSE ("Heater Button")
                    (unwired) ")!" ("string")
                    (unwired) ")" ("string")
                    w3206 = dbl[] [] ("History Data")
                    w3212 = "\r"
                    # "C:\\WinDucom\\Data\\"
                    # "C:\\LAB-IQ-NXT\\data"
                    n2138 = local write "Humidity ( %RH )"(w3194) -> ()
                    n2139 = local write "Frequency ( Hz )"(w3194) -> ()
                    n2140 = local write "Stroke 3"(w3194) -> ()
                    n2141 = local write "speedop"(0.0 ("PIDclk 2")) -> ()
                    n2142 = local write "Set Temp 2"(65.0 ("Set Temp 2")) -> ()
                    n2143 = local write "AIR TEMP"(w3194) -> ()
                    n2144 = local write "clk"(0.0 ("clk")) -> ()
                    n2145 = local write "Stroke 4"(w3194) -> ()
                    n2146 = local write "COF 2"(w3194) -> ()
                    n2147 = local write "TEMP"(w3194) -> ()
                    n2148 = local write "ecr 3"(w3194) -> ()
                    n2149 = local write "FF 3"(w3194) -> ()
                    n2150 = local write "FF 2"(w3194) -> ()
                    n2151 = property on="Humidity ( %RH )" class="WFChart (strict)"("History Data"=w3206) -> ()  [unwired: 2 in, 2 out]
                    n2152 = property on="Coefficient of Friction" class="WFChart (strict)"("History Data"=w3206) -> ()  [unwired: 2 in, 2 out]
                    n2153 = property on="Coefficient of Friction" class="WFChart (strict)"("History Data"=w3206) -> ()  [unwired: 2 in, 2 out]
                    n2154 = property on="Frictional Force ( N )" class="WFChart (strict)"("History Data"=w3206) -> ()  [unwired: 2 in, 2 out]
                    n2155 = property on="Electrical Contact Resistance ( % )" class="WFChart (strict)"("History Data"=w3206) -> ()  [unwired: 2 in, 2 out]
                    n2156 = property on="Electrical Contact Resistance ( % )" class="WFChart (strict)"("History Data"=w3206) -> ()  [unwired: 2 in, 2 out]
                    n2157 = property on="Temperature ( Deg C )" class="WFChart (strict)"("History Data"=w3206) -> ()  [unwired: 2 in, 2 out]
                    n2158 = property on="Frictional Force ( N )" class="WFChart (strict)"("History Data"=w3206) -> ()  [unwired: 2 in, 2 out]
                    n2159 = property on="Coefficient of Friction" class="WFChart (strict)"("History Data"=w3206) -> ()  [unwired: 2 in, 2 out]
                    n2160 = property on="Frictional Force ( N )" class="WFChart (strict)"("History Data"=w3206) -> ()  [unwired: 2 in, 2 out]
                    n2161 = property on="Electrical Contact Resistance ( % )" class="WFChart (strict)"("History Data"=w3206) -> ()  [unwired: 2 in, 2 out]
                    n2162 = property on="Temperature ( Deg C )" class="WFChart (strict)"("History Data"=w3206) -> ()  [unwired: 2 in, 2 out]
                    n2163 = property on="Humidity ( %RH )" class="WFChart (strict)"("History Data"=w3206) -> ()  [unwired: 2 in, 2 out]
                    n2164 = property on="Stroke ( mm )" class="WFChart (strict)"("History Data"=w3207) -> ()  [unwired: 2 in, 2 out]
                    n2165 = property on="Stroke ( mm )" class="WFChart (strict)"("History Data"=w3207) -> ()  [unwired: 2 in, 2 out]
                    n2166 = local write "Humidity"(w3208) -> ()
                    n2167 = local write "Heater Button"(w3208) -> ()
                    n2168 = local read "FILE"() -> (w3202:string)
                    n2169 = disable-structure shown="Enabled" {
                      disable-tunnel: [w3247 _] -> w3193
                      frame Enabled {
                        n2170 = local read "NORMAL LOAD"() -> (w3247:dbl)
                      }
                      frame Disabled {
                      }
                    }
                    n2171 = call "file check.vi"("file name in"=w3202) -> ("error out"=w3205:errorcluster, "file name out"=w3199:string)  [unwired: 9 in]
                    n2172 = call "FILE PATH CREATION.vi"("error in"=w3205, "FILE NAME :"=w3199) -> ("FILE OUT"=w3198:path)  [unwired: 8 in, 1 out]
                    n2173 = Concatenate Strings(w3199, ".dgf" ("Substring")) -> (w3204:string)
                    n2174 = Concatenate Strings(w3199, ".duf" ("Substring")) -> (w3200:string)
                    n2175 = Multiply(x=w3193, y=1.0) -> (x*y=w3226:dbl)
                    n2176 = Build Path(base path=w3198, name or relative path=w3204) -> (appended path=w3197:path)
                    n2177 = Build Path(base path=w3198, name or relative path=w3200) -> (appended path=w3196:path)
                    n2178 = Number To Fractional String(number=w3226, width (-)=i16 5, precision (6)=i16 2) -> (F-format string=w3234:string)  [unwired: 1 in]
                    n2179 = local read "Fuel Discription :"() -> (w3222:string)
                    n2180 = local read "Batch Ref Num :"() -> (w3210:string)
                    n2181 = Get Date/Time String(date format (0)=enum16{"short", "long", "abbreviated"}."short") -> (date string=w3245:string, time string=w3242:string)  [unwired: 2 in]
                    n2182 = local read "Remarks :"() -> (w3221:string)
                    n2183 = Concatenate Strings("Load :- " ("Substring"), w3234, " grams ," ("Substring")) -> (w3233:string)
                    n2184 = local read "String 41"() -> (w3213:string)
                    n2185 = Concatenate Strings(w3222) -> (w3223:string)
                    n2186 = Concatenate Strings(w3210) -> (w3209:string)
                    n2187 = Concatenate Strings("tested by") -> (w3217:string)
                    n2188 = Concatenate Strings("(" ("Substring"), w3245, ")" ("Substring"), w3242) -> (w3215:string)
                    "concatenated string" <- w3215
                    n2189 = Concatenate Strings(w3221, "," ("string")) -> (w3220:string)
                    n2190 = Concatenate Strings("  TIME;      COF;       STROKE;     AIR TEMP;  TEMP;  HUMIDITY;  ECR; PID-OUT; FREQUENCY" ("Substring"), "\r") -> (w3229:string)
                    n2191 = Concatenate Strings(w3213, w3212, "Fuel Discription :-" ("Substring"), w3223, w3212, w3233, w3212, "Batch Ref Num :-" ("Substring"), w3209, w3212, " Remarks :- " ("Substring"), w3220, w3212, " Date :- " ("Substring"), w3215, w3212, "Tested By :-" ("Substring"), w3217) -> (w3227:string)
                    "REMARKS" <- w3227
                    n2192 = call <vilib>:"Write Characters To File.vi"("append to file? (new file:F)"=FALSE, "character string"=w3229, "file path (dialog if empty)"=w3197) -> ()  [unwired: 2 in, 1 out]
                    n2193 = call <vilib>:"Write Characters To File.vi"("append to file? (new file:F)"=FALSE, "character string"=w3227, "file path (dialog if empty)"=w3196) -> ()  [unwired: 2 in, 1 out]
                  }
                  frame #2 {
                    n2194 = local write "Cycles elapsed"(0 ("Cycles elapsed")) -> ()
                    n2195 = local write "cyclecount"(0 ("cyclecount")) -> ()
                    n2196 = local write "Save & Continue"(FALSE ("OK")) -> ()
                    n2197 = local write "autostrtflg"(TRUE ("autostrtflg")) -> ()
                    n2198 = local write "Save"(FALSE ("Save")) -> ()
                    n2199 = Get Date/Time In Seconds() -> (seconds since 1Jan1904=w3252:timestamp)
                    n2200 = To Double Precision Float(number=w3252) -> (double precision float=w3251:dbl)
                    n2201 = local write "acq timer"(w3251) -> ()
                    n2202 = One Button Dialog(message="Please ensure sample is mounted properly and machine is ready in all aspects for testing !", button name ("OK")="Ok") -> ()  [unwired: 1 out]
                  }
                  frame #3 {
                    n2203 = stacked-sequence {
                      frame #0 {
                        n2204 = local write "Main Dashboard Buttons"(T1."Dashboard" ("Main Dashboard Buttons")) -> ()
                        n2205 = local write "Main Tab"(T2."Acquire" ("Main Tab")) -> ()
                      }
                      frame #1 {
                        n2206 = local write "EVENT LOG"("" ("EVENT LOG")) -> ()
                      }
                      frame #2 {
                        n2207 = Wait (ms)(milliseconds to wait=u32 50) -> ()  [unwired: 1 out]
                      }
                      frame #3 {
                        n2208 = disable-structure shown="Disabled" {
                          frame Disabled {
                            n2209 = local read "EVENT LOG"() -> (w3264:string)
                            n2210 = call "Event Log.vi"("Content"="Test Details", "EVENT LOG"=w3264) -> ("EVENT LOG"=w3263:string)  [unwired: 8 in, 1 out]
                            n2211 = local write "EVENT LOG"(w3263) -> ()
                          }
                          frame Enabled {
                          }
                        }
                      }
                      frame #4 {
                        n2212 = Wait (ms)(milliseconds to wait=u32 50) -> ()  [unwired: 1 out]
                      }
                      frame #5 {
                        n2213 = local read "FILE"() -> (w3266:string)
                        n2214 = Concatenate Strings("File Name :" ("Content"), w3266) -> (w3267:string)
                        n2215 = local read "EVENT LOG"() -> (w3270:string)
                        n2216 = call "Event Log.vi"("Content"=w3267, "EVENT LOG"=w3270) -> ("EVENT LOG"=w3269:string)  [unwired: 8 in, 1 out]
                        n2217 = local write "EVENT LOG"(w3269) -> ()
                      }
                      frame #6 {
                        n2218 = Wait (ms)(milliseconds to wait=u32 50) -> ()  [unwired: 1 out]
                      }
                      frame #7 {
                        n2219 = local read "Batch Ref Num :"() -> (w3272:string)
                        n2220 = Concatenate Strings("Batch Ref No :" ("Content"), w3272) -> (w3273:string)
                        n2221 = local read "EVENT LOG"() -> (w3276:string)
                        n2222 = call "Event Log.vi"("Content"=w3273, "EVENT LOG"=w3276) -> ("EVENT LOG"=w3275:string)  [unwired: 8 in, 1 out]
                        n2223 = local write "EVENT LOG"(w3275) -> ()
                      }
                      frame #8 {
                        n2224 = Wait (ms)(milliseconds to wait=u32 50) -> ()  [unwired: 1 out]
                      }
                      frame #9 {
                        n2225 = local read "tested by"() -> (w3278:string)
                        n2226 = Concatenate Strings("Tested By :" ("Content"), w3278) -> (w3279:string)
                        n2227 = local read "EVENT LOG"() -> (w3282:string)
                        n2228 = call "Event Log.vi"("Content"=w3279, "EVENT LOG"=w3282) -> ("EVENT LOG"=w3281:string)  [unwired: 8 in, 1 out]
                        n2229 = local write "EVENT LOG"(w3281) -> ()
                      }
                      frame #10 {
                        n2230 = Wait (ms)(milliseconds to wait=u32 50) -> ()  [unwired: 1 out]
                      }
                      frame #11 {
                        n2231 = local read "TEST STANDARD"() -> (w3285:T3)
                        n2232 = case shown="\"ASTM D6079\", Default" w3285 {
                          tunnel: ["ASTM D6079" "ISO 12156" "CEC F-096-A-06" "Custom"] -> w3284
                          frame "ASTM D6079", Default {
                          }
                          frame "ISO 12156" {
                          }
                          frame "CEC F-096-A-06" {
                          }
                          frame "Custom" {
                          }
                        }
                        n2233 = Concatenate Strings("Test Standard :" ("Content"), w3284) -> (w3286:string)
                        n2234 = local read "EVENT LOG"() -> (w3289:string)
                        n2235 = call "Event Log.vi"("Content"=w3286, "EVENT LOG"=w3289) -> ("EVENT LOG"=w3288:string)  [unwired: 8 in, 1 out]
                        n2236 = local write "EVENT LOG"(w3288) -> ()
                      }
                      frame #12 {
                        n2237 = Wait (ms)(milliseconds to wait=u32 50) -> ()  [unwired: 1 out]
                      }
                      frame #13 {
                        n2238 = local read "Fuel Discription :"() -> (w3295:string)
                        n2239 = Concatenate Strings("Fuel Description :" ("Content"), w3295) -> (w3296:string)
                        n2240 = local read "EVENT LOG"() -> (w3299:string)
                        n2241 = call "Event Log.vi"("Content"=w3296, "EVENT LOG"=w3299) -> ("EVENT LOG"=w3298:string)  [unwired: 8 in, 1 out]
                        n2242 = local write "EVENT LOG"(w3298) -> ()
                      }
                      frame #14 {
                        n2243 = Wait (ms)(milliseconds to wait=u32 50) -> ()  [unwired: 1 out]
                      }
                      frame #15 {
                        n2244 = local read "Remarks :"() -> (w3301:string)
                        n2245 = Concatenate Strings("Remarks :" ("Content"), w3301) -> (w3302:string)
                        n2246 = local read "EVENT LOG"() -> (w3305:string)
                        n2247 = call "Event Log.vi"("Content"=w3302, "EVENT LOG"=w3305) -> ("EVENT LOG"=w3304:string)  [unwired: 8 in, 1 out]
                        n2248 = local write "EVENT LOG"(w3304) -> ()
                      }
                      frame #16 {
                        n2249 = Wait (ms)(milliseconds to wait=u32 50) -> ()  [unwired: 1 out]
                      }
                      frame #17 {
                        n2250 = local read "Operator ID"() -> (w3307:string)
                        n2251 = Concatenate Strings("Operator ID :" ("Content"), w3307) -> (w3309:string)
                        n2252 = local read "EVENT LOG"() -> (w3311:string)
                        n2253 = call "Event Log.vi"("Content"=w3309, "EVENT LOG"=w3311) -> ("EVENT LOG"=w3310:string)  [unwired: 8 in, 1 out]
                        n2254 = local write "EVENT LOG"(w3310) -> ()
                      }
                      frame #18 {
                        n2255 = Wait (ms)(milliseconds to wait=u32 50) -> ()  [unwired: 1 out]
                      }
                      frame #19 {
                        n2256 = disable-structure shown="Disabled" {
                          frame Disabled {
                            n2257 = local read "EVENT LOG"() -> (w3315:string)
                            n2258 = call "Event Log.vi"("Content"="Test Parameter", "EVENT LOG"=w3315) -> ("EVENT LOG"=w3314:string)  [unwired: 8 in, 1 out]
                            n2259 = local write "EVENT LOG"(w3314) -> ()
                          }
                          frame Enabled {
                          }
                        }
                      }
                      frame #20 {
                        n2260 = Wait (ms)(milliseconds to wait=u32 50) -> ()  [unwired: 1 out]
                      }
                      frame #21 {
                        n2261 = local read "Set Hz"() -> (w3319:dbl)
                        n2262 = Number To Fractional String(number=w3319, precision (6)=i16 2) -> (F-format string=w3318:string)  [unwired: 2 in]
                        n2263 = Concatenate Strings("Set Frequency [Hz] :" ("Content"), w3318) -> (w3321:string)
                        n2264 = local read "EVENT LOG"() -> (w3323:string)
                        n2265 = call "Event Log.vi"("Content"=w3321, "EVENT LOG"=w3323) -> ("EVENT LOG"=w3322:string)  [unwired: 8 in, 1 out]
                        n2266 = local write "EVENT LOG"(w3322) -> ()
                      }
                      frame #22 {
                        n2267 = Wait (ms)(milliseconds to wait=u32 50) -> ()  [unwired: 1 out]
                      }
                      frame #23 {
                        n2268 = local read "NORMAL LOAD"() -> (w3326:dbl)
                        n2269 = Number To Fractional String(number=w3326, precision (6)=i16 2) -> (F-format string=w3327:string)  [unwired: 2 in]
                        n2270 = Concatenate Strings("Applied Load [grams] :" ("Content"), w3327) -> (w3329:string)
                        n2271 = local read "EVENT LOG"() -> (w3331:string)
                        n2272 = call "Event Log.vi"("Content"=w3329, "EVENT LOG"=w3331) -> ("EVENT LOG"=w3330:string)  [unwired: 8 in, 1 out]
                        n2273 = local write "EVENT LOG"(w3330) -> ()
                      }
                      frame #24 {
                        n2274 = Wait (ms)(milliseconds to wait=u32 50) -> ()  [unwired: 1 out]
                      }
                      frame #25 {
                        n2275 = local read "Set Strk"() -> (w3334:dbl)
                        n2276 = Number To Fractional String(number=w3334, precision (6)=i16 2) -> (F-format string=w3335:string)  [unwired: 2 in]
                        n2277 = Concatenate Strings("Set Stroke [mm] :" ("Content"), w3335) -> (w3337:string)
                        n2278 = local read "EVENT LOG"() -> (w3339:string)
                        n2279 = call "Event Log.vi"("Content"=w3337, "EVENT LOG"=w3339) -> ("EVENT LOG"=w3338:string)  [unwired: 8 in, 1 out]
                        n2280 = local write "EVENT LOG"(w3338) -> ()
                      }
                      frame #26 {
                        n2281 = Wait (ms)(milliseconds to wait=u32 50) -> ()  [unwired: 1 out]
                      }
                      frame #27 {
